vi "Main_Panel.vi"() -> ()   [LabVIEW 2017]
panel:
  out "Test element":u8(slide) scale=0.0..100.0
  out "Current Time":timestamp
  out "Data Collection Software Path":path
  out "Calibration Software Path":path
  in  "Load Data Collection Software":bool
  in  "Load Calibration Software":bool
  in  "Load VI Manually":path
  in  "Load/Unload":bool
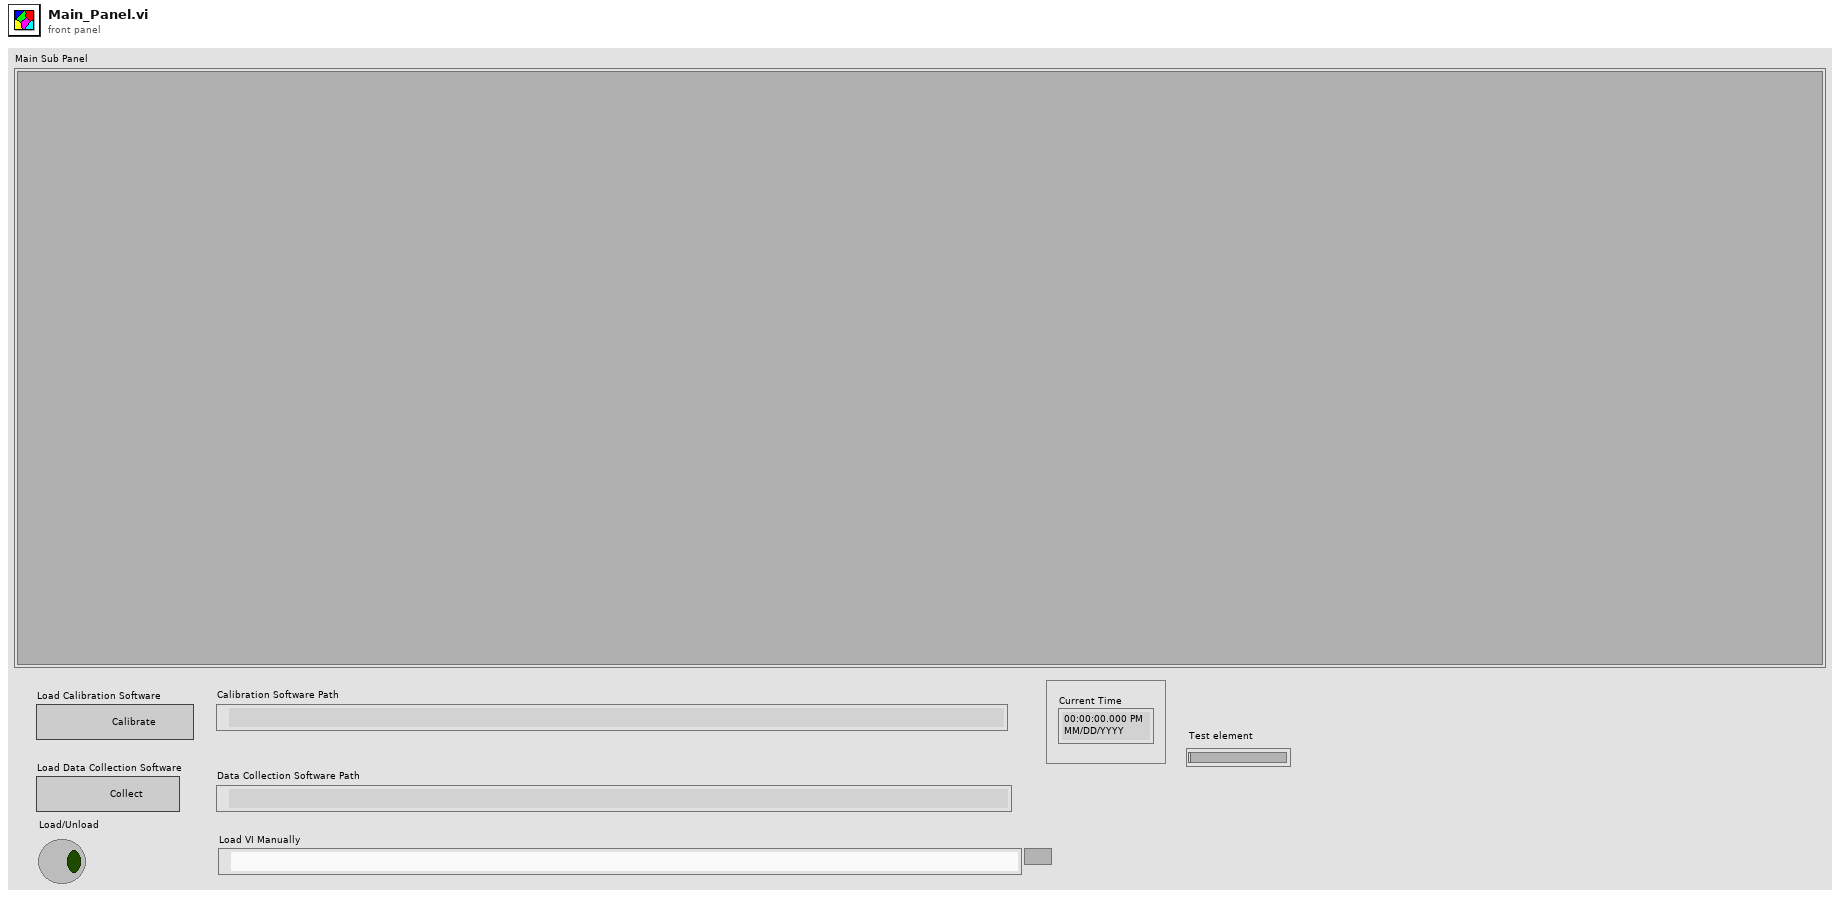
[diagram p1: front panel]
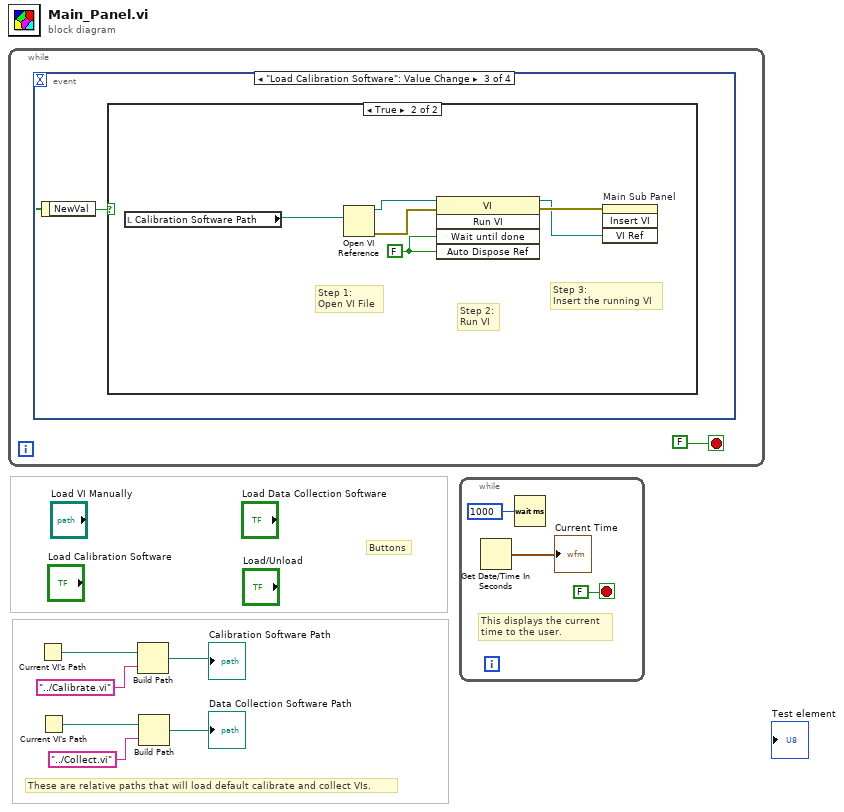
[diagram p0: block diagram]
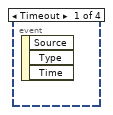
[diagram p2: hidden frame]
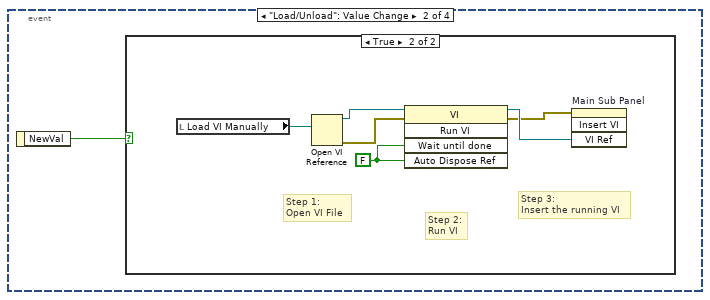
[diagram p3: hidden frame]
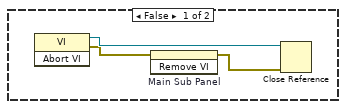
[diagram p4: hidden frame]
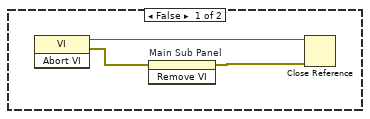
[diagram p5: hidden frame]
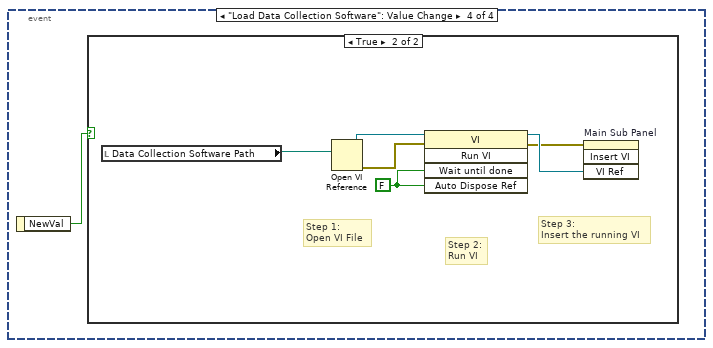
[diagram p6: hidden frame]
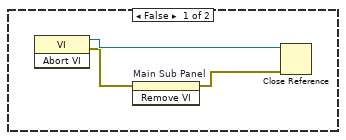
[diagram p7: hidden frame]
diagram:
  # "Buttons"
  # "These are relative paths that will load default calibrate and collect VIs."
  n1 = while {
    stop <- FALSE stop-if-true
    n2 = event shown="[2] \"Load Calibration Software\": Value Change" {
      selector: _ -> [_ _ _ _]
      dyn-events: _ -> [_ _ _ _]
      timeout: _ -> [_ _ _ _]
      event Timeout {
        n3 = event-data() -> ()  [unwired: 1 in, 3 out]
      }
      event "Load/Unload": Value Change {
        n4 = event-data() -> ("NewVal"=w8:bool)  [unwired: 1 in]
        n5 = case shown="True" w8 {
          frame False {
            n6 = invoke class="VI" method="Abort VI"() -> (reference out=w11:refnum<vi>, error out=w10:errorcluster)  [unwired: 3 in, 1 out]
            n7 = invoke on="Main Sub Panel" class="SubPnl" method="Remove VI"(error in=w10) -> (error out=w9:errorcluster)  [unwired: 2 in, 2 out]
            n8 = Close Reference(reference=w11, error in (no error)=w9) -> ()  [unwired: 1 out]
          }
          frame True {
            w15 = FALSE
            # "Step 3:\nInsert the running VI"
            # "Step 2:\nRun VI"
            # "Step 1:\nOpen VI File"
            n9 = local read "Load VI Manually"() -> (w14:path)
            n10 = Open VI Reference(vi path=w14) -> (vi reference=w16:refnum<vi>, error out=w17:errorcluster)  [unwired: 5 in]
            n11 = invoke class="VI" method="Run VI"(reference=w16, error in=w17, "Wait until done"=w15, "Auto Dispose Ref"=w15) -> (reference out=w13:refnum<vi>, error out=w12:errorcluster)  [unwired: 1 in, 3 out]
            n12 = invoke on="Main Sub Panel" class="SubPnl" method="Insert VI"(error in=w12, "VI Ref"=w13) -> ()  [unwired: 2 in, 4 out]
          }
        }
      }
      event "Load Calibration Software": Value Change {
        n13 = event-data() -> ("NewVal"=w18:bool)  [unwired: 1 in]
        n14 = case shown="True" w18 {
          frame False {
            n15 = invoke class="VI" method="Abort VI"() -> (reference out=w21:refnum<vi>, error out=w20:errorcluster)  [unwired: 3 in, 1 out]
            n16 = invoke on="Main Sub Panel" class="SubPnl" method="Remove VI"(error in=w20) -> (error out=w19:errorcluster)  [unwired: 2 in, 2 out]
            n17 = Close Reference(reference=w21, error in (no error)=w19) -> ()  [unwired: 1 out]
          }
          frame True {
            w24 = FALSE
            # "Step 3:\nInsert the running VI"
            # "Step 2:\nRun VI"
            # "Step 1:\nOpen VI File"
            n18 = local read "Calibration Software Path"() -> (w27:path)
            n19 = Open VI Reference(vi path=w27) -> (vi reference=w26:refnum<vi>, error out=w25:errorcluster)  [unwired: 5 in]
            n20 = invoke class="VI" method="Run VI"(reference=w26, error in=w25, "Wait until done"=w24, "Auto Dispose Ref"=w24) -> (reference out=w22:refnum<vi>, error out=w23:errorcluster)  [unwired: 1 in, 3 out]
            n21 = invoke on="Main Sub Panel" class="SubPnl" method="Insert VI"(error in=w23, "VI Ref"=w22) -> ()  [unwired: 2 in, 4 out]
          }
        }
      }
      event "Load Data Collection Software": Value Change {
        n22 = event-data() -> ("NewVal"=w28:bool)  [unwired: 1 in]
        n23 = case shown="True" w28 {
          frame False {
            n24 = invoke class="VI" method="Abort VI"() -> (reference out=w31:refnum<vi>, error out=w29:errorcluster)  [unwired: 3 in, 1 out]
            n25 = invoke on="Main Sub Panel" class="SubPnl" method="Remove VI"(error in=w29) -> (error out=w30:errorcluster)  [unwired: 2 in, 2 out]
            n26 = Close Reference(reference=w31, error in (no error)=w30) -> ()  [unwired: 1 out]
          }
          frame True {
            w34 = FALSE
            # "Step 3:\nInsert the running VI"
            # "Step 2:\nRun VI"
            # "Step 1:\nOpen VI File"
            n27 = local read "Data Collection Software Path"() -> (w37:path)
            n28 = Open VI Reference(vi path=w37) -> (vi reference=w36:refnum<vi>, error out=w35:errorcluster)  [unwired: 5 in]
            n29 = invoke class="VI" method="Run VI"(reference=w36, error in=w35, "Wait until done"=w34, "Auto Dispose Ref"=w34) -> (reference out=w33:refnum<vi>, error out=w32:errorcluster)  [unwired: 1 in, 3 out]
            n30 = invoke on="Main Sub Panel" class="SubPnl" method="Insert VI"(error in=w32, "VI Ref"=w33) -> ()  [unwired: 2 in, 4 out]
          }
        }
      }
    }
  }
  n31 = Current VI's Path() -> (path=w6:path)
  n32 = Current VI's Path() -> (path=w3:path)
  n33 = Build Path(base path=w6, name or relative path="../Calibrate.vi") -> (appended path=→"Calibration Software Path":path)
  n34 = Build Path(base path=w3, name or relative path="../Collect.vi") -> (appended path=→"Data Collection Software Path":path)
  n35 = while {
    stop <- FALSE stop-if-true
    # "This displays the current\ntime to the user."
    n36 = Get Date/Time In Seconds() -> (seconds since 1Jan1904=→"Current Time":timestamp)
    n37 = Wait (ms)(milliseconds to wait=u32 1000) -> ()  [unwired: 1 out]
  }
